vi "Auto Update Step Result in UI Control.vi"(4 "Step No":i32, 5 "Data Cluster in":T1, 7 "Test List":refnum<vi>, 8 "Acutal(T)/Reset(F)?":bool, 9 "Reset_SEQ":string[][](array[string]), 10 "Step Result":string[][](array[string]), 11 "Boolean in":refnum<vi>) -> (3 "Data Cluster out":T1)   [LabVIEW 2020]
uses:
  controls/Auto UI Data.ctl
  controls/Configuration Details.ctl
  <vilib>/Utility/miscctls.llb/LVRowAndColumnTypeDef.ctl
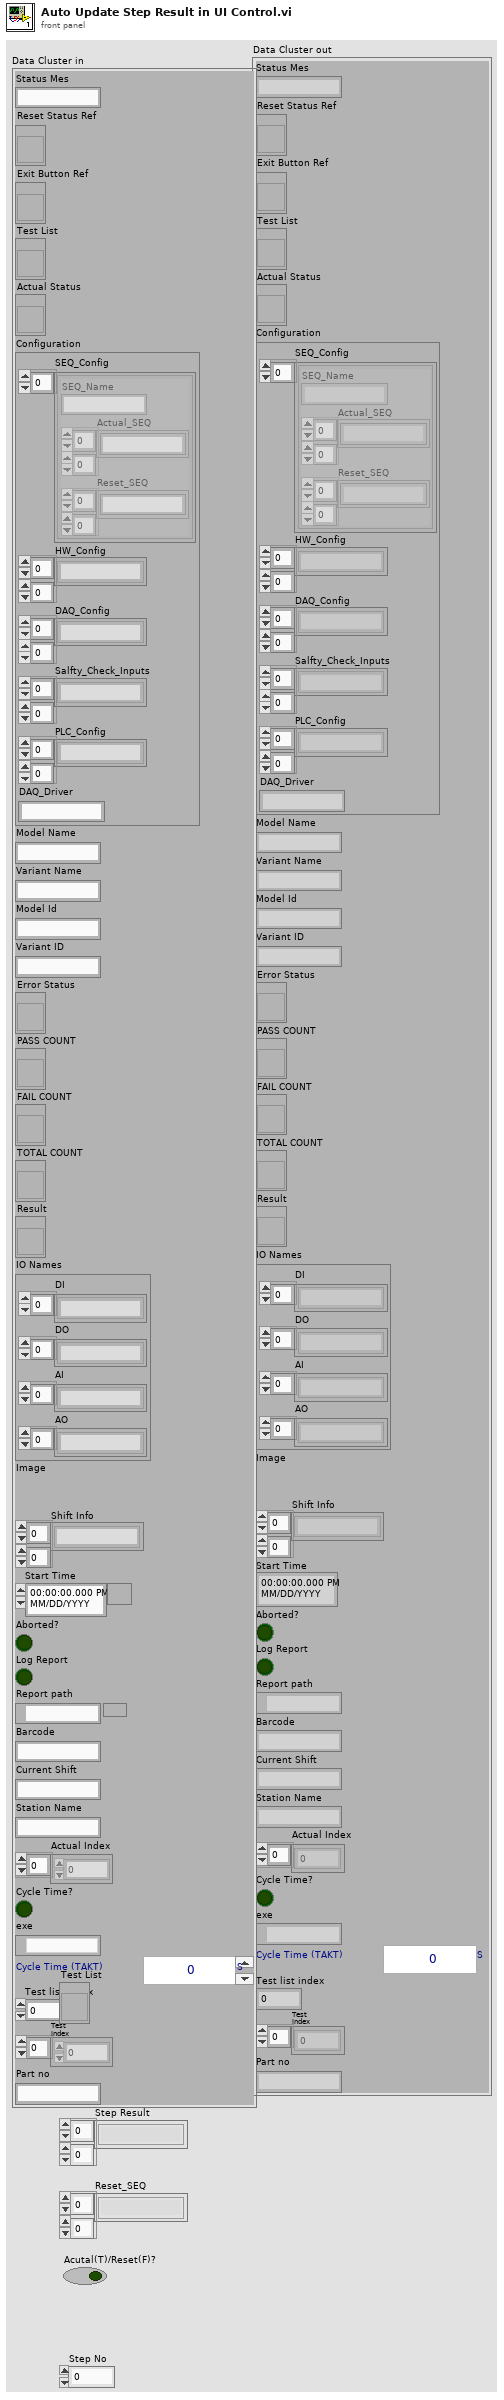
[diagram p1: front panel]
types:
  T1 = typedef "Auto UI Data.ctl" = cluster{"Status Mes":string, "Reset Status Ref":refnum<vi>, "Exit Button Ref":refnum<vi>, "Test List":refnum<vi>, "Actual Status":refnum<vi>, "Configuration":T2, "Model Name":string, "Variant Name":string, "Model Id":string, "Variant ID":string, "Error Status":refnum<vi>, "PASS COUNT":refnum<vi>, "FAIL COUNT":refnum<vi>, "TOTAL COUNT":refnum<vi>, "Result":refnum<vi>, "IO Names":cluster{"DI":string[], "DO":string[], "AI":string[], "AO":string[]}, "Image":T3, "Shift Info":string[][], "Start Time":timestamp, "Aborted?":bool, "Log Report":bool, "Report path":path, "Barcode":string, "Current Shift":string, "Station Name":string, "Actual Index":i32[], "Cycle Time?":bool, "exe":path, "Cycle Time (TAKT)":u16, "Test list index":u32, "Test index":u32[], "Part no":string}
  T2 = typedef "Configuration Details.ctl" = cluster{"SEQ_Config":cluster{"SEQ_Name":string, "Actual_SEQ":string[][], "Reset_SEQ":string[][]}[], "HW_Config":string[][], "DAQ_Config":string[][], "Salfty_Check_Inputs":string[][], "PLC_Config":string[][], "DAQ_Driver":string}
  T3 = typedef "IMAQ Image.ctl" = refnum<image>
  T4 = enum8{"Enabled", "Disabled", "Disabled and Grayed Out"}
  T5 = typedef "LVRowAndColumnTypeDef.ctl" = cluster{"Row":i32, "Column":i32}
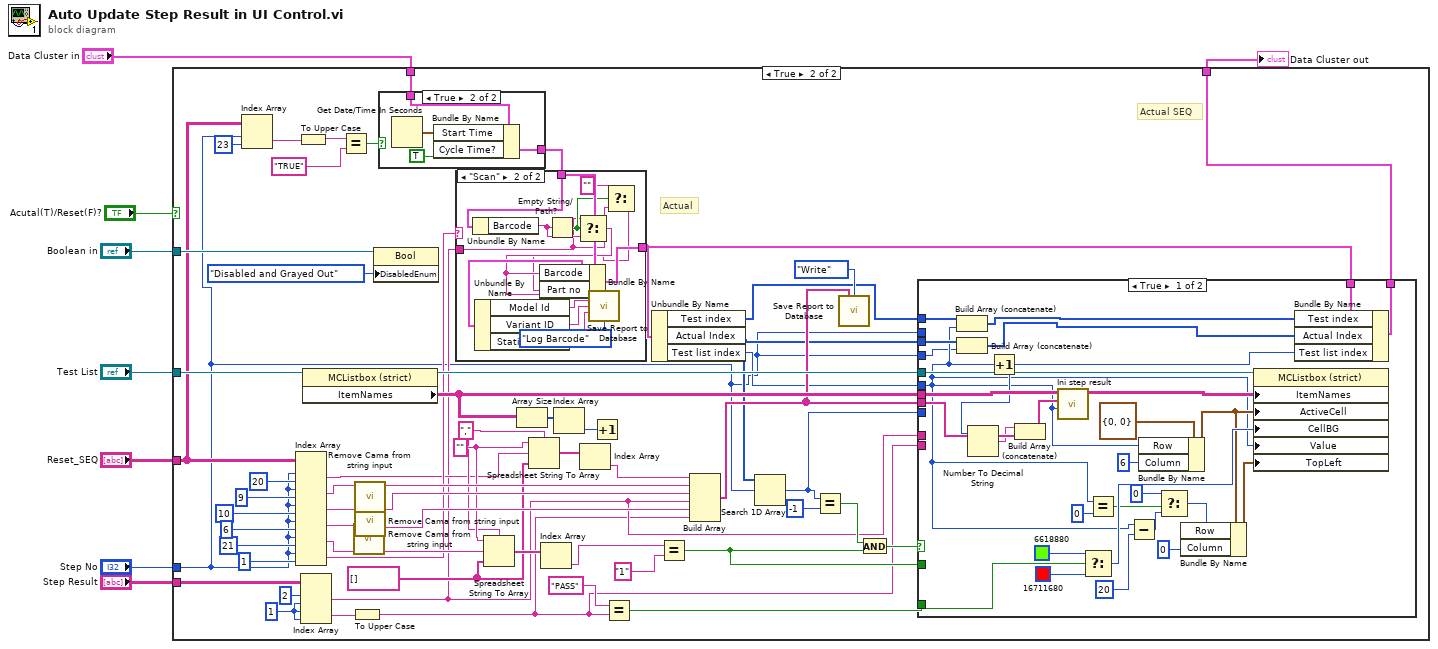
[diagram p0: block diagram]
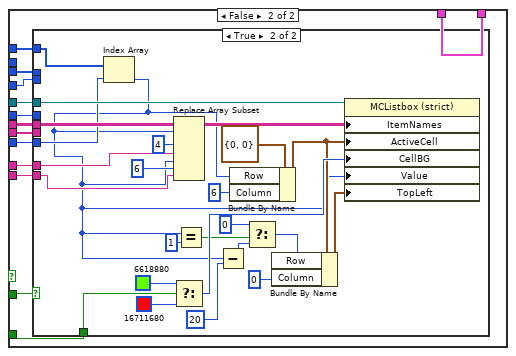
[diagram p5: hidden frame]
diagram:
  n1 = case shown="True" "Acutal(T)/Reset(F)?" {
    tunnel: "Step No" -> [_ w12]
    tunnel: "Step Result" -> [_ w67]
    tunnel: "Test List" -> [_ w66]
    tunnel: "Reset_SEQ" -> [_ w24]
    tunnel: [w9 w33] -> w7
    tunnel: "Data Cluster in" -> [w9 w18]
    tunnel: "Boolean in" -> [_ w43]
    frame False {
      # "Reset SEQ"
    }
    frame True {
      w37 = "," ("delimiter (Tab)")
      w38 = "" ("format string")
      w39 = string[] [] ("appended array")
      w57 = 1 ("index (row)")
      # "Actual SEQ"
      # "Actual"
      n2 = Index Array(array=w24, index (row)=w12, index (col)=23 ("disabled index (col)")) -> (element=w22:string)
      n3 = Index Array(array=w24, index (row) #1=w12, index (col) #1=20 ("disabled index (col)"), index (row) #2=w12, index (col) #2=9 ("disabled index (col)"), index (row) #3=w12, index (col) #3=10 ("disabled index (col)"), index (row) #4=w12, index (col) #4=6 ("disabled index (col)"), index (row) #5=w12, index (col) #5=21 ("index (row)"), index (row) #6=w12, index (col) #6=1 ("disabled index (col)")) -> (element #1=w35:string, element #2=w62:string, element #3=w61:string, element #4=w51:string, element #5=w46:string, element #6=w44:string)
      n4 = To Upper Case(1:w22) -> (0:w21:string)
      n5 = Index Array(array=w67, index (row) #1=2 ("index (row)"), index (col) #1=w57, index (row) #2=w57, index (col) #2=w57) -> (element #1=w26:string, element #2=w56:string)
      n6 = property class="MCListbox (strict)"(reference=w66) -> (reference out=w58:refnum<vi>, "ItemNames"=w59:string[][])  [unwired: 1 in, 1 out]
      n7 = Equal?(x=w21, y="TRUE") -> (x = y?=w19:bool)
      n8 = To Upper Case(1:w56) -> (0:w25:string)
      n9 = call "Remove Cama from string input.vi"("String in"=w51) -> ("string out"=w50:string)  [unwired: 10 in]
      n10 = call "Remove Cama from string input.vi"("String in"=w62) -> ("string out"=w55:string)  [unwired: 10 in]
      n11 = call "Remove Cama from string input.vi"("String in"=w61) -> ("string out"=w54:string)  [unwired: 10 in]
      n12 = property class="Bool"(reference=w43, "DisabledEnum"=T4."Disabled and Grayed Out" ("Disabled")) -> ()  [unwired: 1 in, 2 out]
      n13 = case shown="True" w19 {
        tunnel: [w69 w72] -> w17
        tunnel: w18 -> [w69 w73]
        frame False {
        }
        frame True {
          n14 = Get Date/Time In Seconds() -> (seconds since 1Jan1904=w71:timestamp)
          n15 = Bundle By Name(cluster=w73, "Start Time"=w71, "Cycle Time?"=TRUE) -> (w72:T1)
        }
      }
      n16 = case shown="\"Scan\"" w44 {
        tunnel: w17 -> [w74 w81]
        tunnel: [w74 w86] -> w32
        tunnel: w26 -> [_ w77]
        frame Default {
        }
        frame "Scan" {
          n17 = Unbundle By Name(w81) -> ("Barcode"=w79:string)
          n18 = Empty String/Path?(string/path=w79) -> (empty?=w78:bool)
          n19 = Select(t=w77, s=w78, f=w79) -> (s? t:f=w80:string)
          n20 = Select(t="", s=w78, f=w77) -> (s? t:f=w76:string)
          n21 = Bundle By Name(cluster=w81, "Barcode"=w80, "Part no"=w76) -> (w86:T1)
          n22 = Unbundle By Name(w86) -> ("Model Id"=w85:string, "Variant ID"=w84:string, "Station Name"=w82:string)
          n23 = call "Save Report to Database.vi"("barcode"=w80, "Option"=enum16{"Write", "Log", "Log Barcode"}."Log Barcode", "modelid"=w85, "varintid"=w84, "stationid"=w82) -> ()  [unwired: 10 in, 1 out]
        }
      }
      n24 = Spreadsheet String To Array(delimiter (Tab)=w37, format string=w38, spreadsheet string=w46, array type (2D Dbl)=w39) -> (array=w41:string[])
      n25 = Array Size(array=w59) -> (size(s)=w68:i32[])
      n26 = Spreadsheet String To Array(delimiter (Tab)=w37, format string=w38, spreadsheet string=w35, array type (2D Dbl)=w39) -> (array=w36:string[])
      n27 = Index Array(array=w41) -> (element=w40:string)  [unwired: 1 in]
      n28 = Index Array(array=w68) -> (element=w49:i32)  [unwired: 1 in]
      n29 = Index Array(array=w36) -> (element=w34:string)  [unwired: 1 in]
      n30 = Increment(x=w49) -> ()  [unwired: 1 out]
      n31 = Equal?(x="PASS", y=w25) -> (x = y?=w53:bool)
      n32 = Unbundle By Name(w32) -> ("Test index"=w11:u32[], "Actual Index"=w14:i32[], "Test list index"=w13:u32)
      n33 = Equal?(x=w40, y="1") -> (x = y?=w28:bool)
      n34 = Build Array(w34, w55, w54, w26, w50, w25) -> (w16:string[])
      n35 = Search 1D Array(1D array=w14, element=w12) -> (index of element=w10:i32)  [unwired: 1 in]
      n36 = Equal?(x=w10, y=-1) -> (x = y?=w29:bool)
      n37 = call "Save Report to Database.vi"("Input"=w16, "Option"=enum16{"Write", "Log", "Log Barcode"}."Write") -> ()  [unwired: 13 in, 1 out]
      n38 = And(x=w29, y=w28) -> (x .and. y?=w30:bool)
      n39 = case shown="True" w30 {
        tunnel: w16 -> [w95 w129]
        tunnel: w59 -> [w97 w128]
        tunnel: w58 -> [w116 w127]
        tunnel: w53 -> [w113 w126]
        tunnel: [w104 w123] -> w33
        tunnel: w32 -> [w105 w123]
        tunnel: w14 -> [w103 w125]
        tunnel: w12 -> [w87 w124]
        tunnel: w28 -> [_ w121]
        tunnel: w25 -> [_ w122]
        tunnel: w26 -> [_ w120]
        tunnel: w13 -> [w90 w119]
        tunnel: w12 -> [_ _]
        tunnel: w11 -> [w91 w117]
        tunnel: w10 -> [_ w118]
        frame True {
          n40 = Build Array (concatenate)(w91, w90) -> (w89:u32[])
          n41 = Build Array (concatenate)(w103, w87) -> (w88:i32[])
          n42 = Increment(x=w90) -> (x+1=w93:u32)
          n43 = Number To Decimal String(number=w93) -> (decimal integer string=w92:string)  [unwired: 1 in]
          n44 = Build Array (concatenate)(w92, w95) -> (w94:string[])
          n45 = call "Ini step result.vi"("index (row)"=w90, "new element/subarray"=w94, "Out Data"=w97) -> ("output array"=w96:string[][])  [unwired: 8 in]
          n46 = Select(t=u32 6618880, s=w113, f=u32 16711680) -> (s? t:f=w110:u32)
          n47 = Equal?(x=w90, y=0) -> (x = y?=w102:bool)
          n48 = Subtract(x=w90, y=20) -> (x-y=w101:u32)
          n49 = Bundle By Name(cluster=T5 {"Row"=0, "Column"=0} ("Active Cell:Active Cell"), "Row"=w90, "Column"=6) -> (w109:T5)
          n50 = Select(t=0, s=w102, f=w101) -> (s? t:f=w100:u32)
          n51 = Bundle By Name(cluster=w109, "Row"=w100, "Column"=0) -> (w108:T5)
          n52 = property class="MCListbox (strict)"(reference=w116, "ItemNames"=w96, "ActiveCell"=w109, "CellBG"=w110, "Value"=w90, "TopLeft"=w108) -> ()  [unwired: 1 in, 2 out]
          n53 = Bundle By Name(cluster=w105, "Test index"=w89, "Actual Index"=w88, "Test list index"=w93) -> (w104:T1)
        }
        frame False {
          n54 = case shown="True" w121 {
            tunnel: w129 -> [_ _]
            tunnel: w128 -> [_ w154]
            tunnel: w127 -> [_ w153]
            tunnel: w126 -> [_ w149]
            tunnel: w125 -> [_ _]
            tunnel: w124 -> [_ _]
            tunnel: w122 -> [_ w138]
            tunnel: w120 -> [_ w140]
            tunnel: w119 -> [_ _]
            tunnel: w118 -> [_ w132]
            tunnel: w117 -> [_ w131]
            frame False {
            }
            frame True {
              n55 = Index Array(array=w131, index=w132) -> (element=w130:u32)
              n56 = Replace Array Subset(array=w154, new element #1=w140, index (row) #1=w130, index (col) #1=4 ("disabled index (col)"), new element #2=w138, index (row) #2=w130, index (col) #2=6 ("disabled index (col)")) -> (w152:string[][])
              n57 = Select(t=u32 6618880, s=w149, f=u32 16711680) -> (s? t:f=w146:u32)
              n58 = Equal?(x=w130, y=1) -> (x = y?=w136:bool)
              n59 = Subtract(x=w130, y=20) -> (x-y=w135:u32)
              n60 = Bundle By Name(cluster=T5 {"Row"=0, "Column"=0} ("Active Cell:Active Cell"), "Row"=w130, "Column"=6) -> (w145:T5)
              n61 = Select(t=0, s=w136, f=w135) -> (s? t:f=w134:u32)
              n62 = Bundle By Name(cluster=w145, "Row"=w134, "Column"=0) -> (w144:T5)
              n63 = property class="MCListbox (strict)"(reference=w153, "ItemNames"=w152, "ActiveCell"=w145, "CellBG"=w146, "Value"=w130, "TopLeft"=w144) -> ()  [unwired: 1 in, 2 out]
            }
          }
        }
      }
    }
  }
  "Data Cluster out" <- w7
